vi "Output_channels.vi"(10 "?":dbl, 11 "nchan":u32) -> (0 "error out":errorcluster, 3 "Refnum out":refnum<k21>)   [LabVIEW 2021]
uses:
  <vilib>/DAQmx/create/channels.llb/DAQmx Create Channel (AO-Voltage-Basic).vi
panel:
  out "Numeric Control":i32
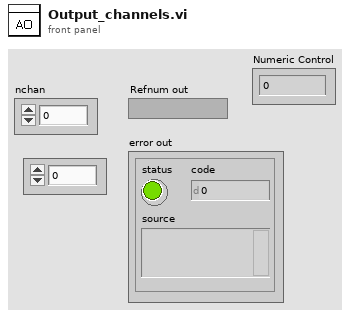
[diagram p1: front panel]
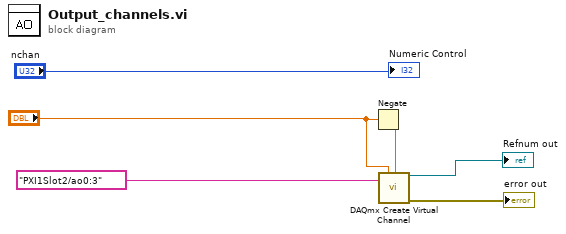
[diagram p0: block diagram]
diagram:
  n1 = Negate(x="?") -> (-x=w1:dbl)
  n2 = call-poly <vilib>:"DAQmx Create Virtual Channel.vi"("maximum value"="?", "minimum value"=w1, "physical channels"=tag "PXI1Slot2/ao0:3") -> ("task out"=→"Refnum out":refnum<k21>, "error out"=→"error out":errorcluster)  [unwired: 11 in]
  "Numeric Control" <- "nchan"
